vi "Authorization log.vi"(6 "EXTRA":string, 8 "EXPIRE":timestamp, 9 "SN":string, 10 "CUSTOMER":string, 11 "hw ID":string) -> (3 "concatenated string":string)   [LabVIEW 2011]
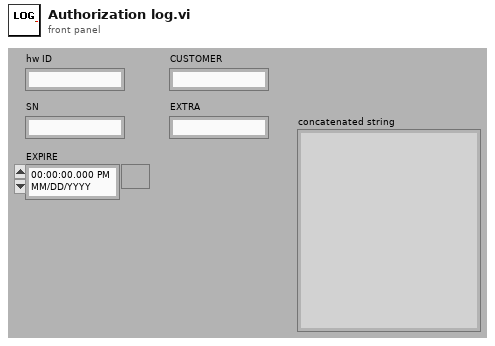
[diagram p1: front panel]
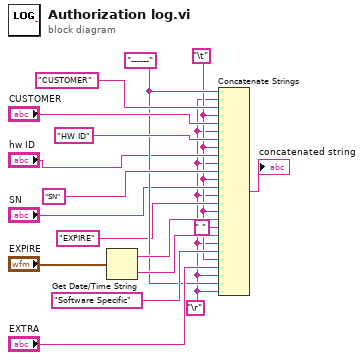
[diagram p0: block diagram]
diagram:
  w8 = "------" ("string")
  w2 = "\r"
  w3 = "\t"
  n1 = Get Date/Time String(seconds (now)="EXPIRE") -> (date string=w12:string, time string=w11:string)  [unwired: 2 in]
  n2 = Concatenate Strings(w8, w2, "CUSTOMER" ("string"), w3, "CUSTOMER", w2, "HW ID" ("string"), w3, "hw ID", w2, "SN" ("string"), w3, "SN", w2, "EXPIRE" ("string"), w3, w12, " " ("string"), w11, w2, "Software Specific" ("string"), w3, "EXTRA", w2, w8, w2) -> (→"concatenated string":string)
